vi "Teste.vi"(9 "type specifier VI Refnum (for type only) 2":refnum<vi>, 11 "vi path":path) -> ()   [LabVIEW 2022 SP3, in "Phoenix.lvclass"]
uses:
  Phoenix.lvclass
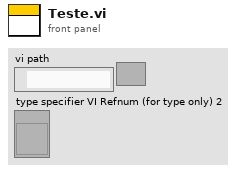
[diagram p1: front panel]
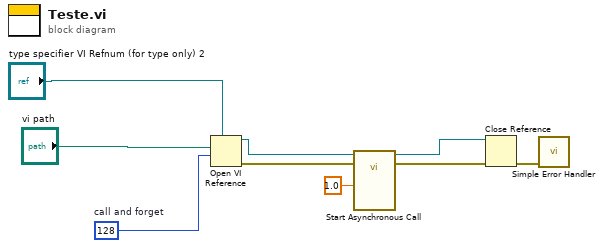
[diagram p0: block diagram]
diagram:
  w9 = 128  # call and forget
  n1 = Open VI Reference(type specifier VI Refnum (for type only)="type specifier VI Refnum (for type only) 2", vi path="vi path", options=w9) -> (vi reference=w1:refnum<vi>, error out=w8:errorcluster)  [unwired: 3 in]
  n2 = call-by-ref "Start Asynchronous Call"(reference=w1, error in=w8, "FPS"=1.0) -> (reference out=w6:refnum<vi>, error out=w7:errorcluster)  [unwired: 11 in]
  n3 = Close Reference(reference=w6, error in (no error)=w7) -> (error out=w5:errorcluster)
  n4 = call <vilib>:"Simple Error Handler.vi"("error in (no error)"=w5) -> ()  [unwired: 4 in, 5 out]
